vi "FormatForDisplay_TeamStats (SubVI).vi"(11 "SR Data":T2[](array[typedef])) -> (3 "DisplayFormat":T1[](array[typedef]) {"Open SRs" scale=0.0..40.0; "Solved in more then 5 Workdays" scale=0.0..40.0; "In Work SRs" scale=0.0..40.0; "Solved Within 5 workdays" scale=0.0..40.0; "New SRs" scale=0.0..40.0})   [LabVIEW 2017]
uses:
  TypeDefs/Weekly_SR_Stats.ctl
  MainFrame/TypeDefs/DisplayCluster.ctl
  DS_Lib.lvlib
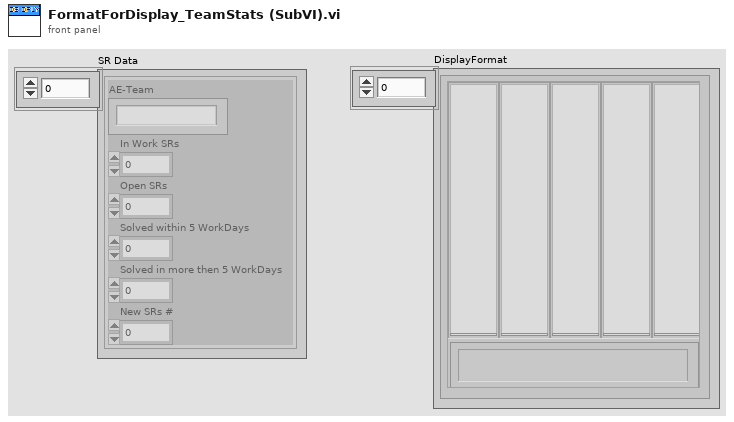
[diagram p1: front panel]
types:
  T1 = typedef "DS_Lib.lvlib/DisplayCluster.ctl" = cluster{"New SRs":u8, "Solved Within 5 workdays":u8, "In Work SRs":u8, "Solved in more then 5 Workdays":u8, "Open SRs":u8, "AE-Team":string}
  T2 = typedef "DS_Lib.lvlib/Weekly_SR_Stats.ctl" = cluster{"AE-Team":string, "In Work SRs":i32, "Open SRs":i32, "Solved within 5 WorkDays":i32, "Solved in more then 5 WorkDays":i32, "New SRs #":i32}
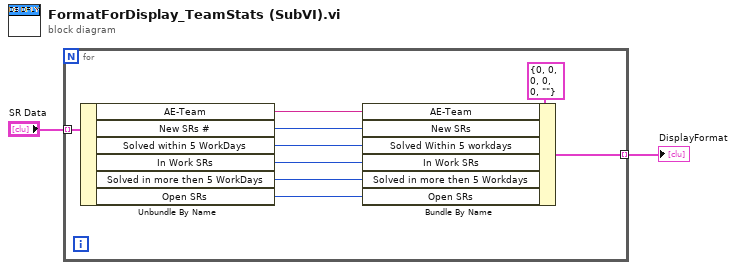
[diagram p0: block diagram]
diagram:
  n1 = for {
    tunnel: "SR Data" -> [w11] mode=indexing
    tunnel: [w4] -> w1 mode=indexing
    n2 = Unbundle By Name(w11) -> ("AE-Team"=w3:string, "New SRs #"=w9:i32, "Solved within 5 WorkDays"=w8:i32, "In Work SRs"=w7:i32, "Solved in more then 5 WorkDays"=w6:i32, "Open SRs"=w5:i32)
    n3 = Bundle By Name(cluster=T1 {"New SRs"=0, "Solved Within 5 workdays"=0, "In Work SRs"=0, "Solved in more then 5 Workdays"=0, "Open SRs"=0, "AE-Team"=""} ("Team"), "AE-Team"=w3, "New SRs"=w9, "Solved Within 5 workdays"=w8, "In Work SRs"=w7, "Solved in more then 5 Workdays"=w6, "Open SRs"=w5) -> (w4:T1)
  }
  "DisplayFormat" <- w1
